vi "ADIS16448 Loop.vi"(8 "error in":errorcluster) -> ()   [LabVIEW 2019]
uses:
  Typedef/ADIS16448 Device Reference.ctl
  Typedef/ADIS16448 Hardware Configuration.ctl
  <vilib>/Rock Robotics/WPI/SPI/WPI_SPIMode.ctl
  <vilib>/Rock Robotics/SystemInterfaces/DIO/FPGA_DIOChannel.ctl
  <vilib>/Rock Robotics/SystemInterfaces/spilib/spi_bus.ctl
  Typedef/ADIS16448 Status.ctl
  Typedef/ADIS16448 Process.ctl
  Typedef/ADIS16448 Command Type.ctl
  <vilib>/Rock Robotics/SystemInterfaces/CounterEncoderSourceConvertion/FPGA_CounterEncoderSourceConvertionLVSourceType.ctl
  <vilib>/Rock Robotics/SystemInterfaces/DIO/FPGA_DIODigitalSourceChannel.ctl
  <vilib>/Rock Robotics/SystemInterfaces/AnalogTrigger/FPGA_AnalogTriggerIndex.ctl
  <vilib>/Rock Robotics/SystemInterfaces/AnalogTrigger/FPGA_AnalogTriggerOutType.ctl
  <vilib>/Rock Robotics/WPI/SPI/WPI_SPIDevRef.ctl
  Typedef/ADIS16448 Data.ctl
  Typedef/ADIS16448 Register.ctl
  <vilib>/Rock Robotics/WPI/Counter/WPI_CounterDigitalInputToDigitalSource.vi
panel:
  in  "Calibration Time":i32
  in  "ADIS16448DevRef":T1={"DevStatus"={"status"=FALSE, "code"=0, "source"=""}, "Hardware Config"={"SPI Clock Rate (Hz)"=1000000.0, "IMU SPI Mode (3)"=enum."Mode 3 (Clk Idle High,Sample on Trailing)", "IMU Reset Pin"=enum."SPI Port CS2", "IMU SPI Bus"=enum."SPI On-Board, CS0", "IMU Data Ready Pin"=enum."SPI Port CS1", "Stall Config"={"Pow2BytesPerRead"=255, "StallTicks"=640, "CsToSclkTicks"=5}, "IMU Status LED Pin"=enum."DIO MXP 9"}, "Calibration Complete"=refnum, "Last Value Reference"=refnum, "Sychronous Process VI"=refnum, "Cmd FIFO"=refnum, "Source"={"DevStatus"={"status"=FALSE, "code"=0, "source"=""}, "AnalogTriggerMode?"=FALSE, "DigitalMode"={"DIO Channel"=enum."Disabled"}, "AnalogTriggerMode"={"AnalogTriggerIndex"=enum."Trig 0", "OutputType"=enum."InWindow"}}, "IMU Status LED Pin"=enum."DIO MXP 9", "Calibration Time"=5}
  in  "Main Name":string
  # "I need to skip the first 6 points.\nDon't use pt-bt-pt to calc avg.\nPublish DC and RMS and CRC errors.\nAdd subVI to recalibrate.\nAdd back the Fuzing code"
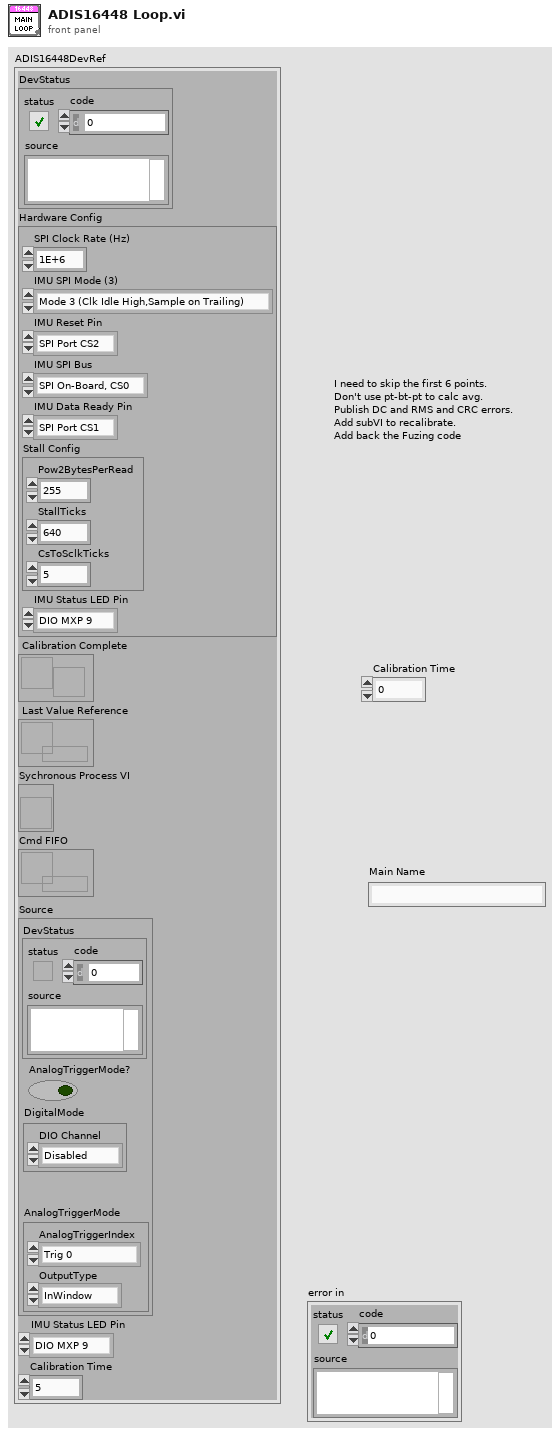
[diagram p1: front panel]
types:
  T1 = typedef "ADIS16448 Device Reference.ctl" = cluster{"DevStatus":errorcluster, "Hardware Config":T2, "Calibration Complete":refnum<notifier>, "Last Value Reference":refnum<data-value>, "Sychronous Process VI":T6, "Cmd FIFO":refnum<k33>, "Source":T7, "IMU Status LED Pin":T4, "Calibration Time":u32}
  T2 = typedef "ADIS16448 Hardware Configuration.ctl" = cluster{"SPI Clock Rate (Hz)":dbl, "IMU SPI Mode (3)":T3, "IMU Reset Pin":T4, "IMU SPI Bus":T5, "IMU Data Ready Pin":T4, "Stall Config":cluster{"Pow2BytesPerRead":u8, "StallTicks":u16, "CsToSclkTicks":u8}, "IMU Status LED Pin":T4}
  T3 = typedef "WPI_SPIMode.ctl" = enum16{"Mode 0 (Clk Idle Low,Sample on Leading)", "Mode 1 (Clk Idle Low,Sample on Trailing)", "Mode 2 (Clk Idle High,Sample on Leading)", "Mode 3 (Clk Idle High,Sample on Trailing)"}
  T4 = typedef "FPGA_DIOChannel.ctl" = enum8{"DIO 0", "DIO 1", "DIO 2", "DIO 3", "DIO 4", "DIO 5", "DIO 6", "DIO 7", "DIO 8", "DIO 9", "DIO MXP 0", "DIO MXP 1", "DIO MXP 2", "DIO MXP 3", "DIO MXP 4", "DIO MXP 5", "DIO MXP 6", "DIO MXP 7", "DIO MXP 8", "DIO MXP 9", "DIO MXP 10", "DIO MXP 11", "DIO MXP 12", "DIO MXP 13", "DIO MXP 14", "DIO MXP 15", "SPI Port CS1", "SPI Port CS2", "SPI Port CS3", "SPI Port MISO", "SPI Port MOSI", "Invalid"}
  T5 = typedef "spi_bus.ctl" = enum16{"SPI On-Board, CS0", "SPI On-Board, CS1", "SPI On-Board, CS2", "SPI On-Board, CS3", "SPI MXP", "Invalid"}
  T6 = typedef "ADIS16448 Process.ctl" = refnum<vi>
  T7 = typedef "FPGA_CounterEncoderSourceConvertionLVSourceType.ctl" = cluster{"DevStatus":errorcluster, "AnalogTriggerMode?":bool, "DigitalMode":cluster{"DIO Channel":T8}, "AnalogTriggerMode":cluster{"AnalogTriggerIndex":T9, "OutputType":T10}}
  T8 = typedef "FPGA_DIODigitalSourceChannel.ctl" = enum8{"DIO 0", "DIO 1", "DIO 2", "DIO 3", "DIO 4", "DIO 5", "DIO 6", "DIO 7", "DIO 8", "DIO 9", "DIO MXP 0", "DIO MXP 1", "DIO MXP 2", "DIO MXP 3", "DIO MXP 4", "DIO MXP 5", "DIO MXP 6", "DIO MXP 7", "DIO MXP 8", "DIO MXP 9", "DIO MXP 10", "DIO MXP 11", "DIO MXP 12", "DIO MXP 13", "DIO MXP 14", "DIO MXP 15", "SPI Port CS1", "SPI Port CS2", "SPI Port CS3", "SPI Port MISO", "SPI Port MOSI", "Disabled"}
  T9 = typedef "FPGA_AnalogTriggerIndex.ctl" = enum8{"Trig 0", "Trig 1", "Trig 2", "Trig 3", "Trig 4", "Trig 5", "Trig 6", "Trig 7", "Invalid"}
  T10 = typedef "FPGA_AnalogTriggerOutType.ctl" = enum16{"InWindow", "TriggerState", "Rising", "Falling"}
  T11 = cluster{"Gyro X":dbl, "Gyro Y":dbl, "Gyro Z":dbl}[]
  T12 = typedef "WPI_SPIDevRef.ctl" = cluster{"DevStatus":errorcluster, "Handle":i32, "SPI Bus":T5}
  T13 = cluster{"SPIDevRef":T12, "Data Counter":u16, "Digital Source":T7, "Bytes Per Sample":u32, "ADIS16448DevRef":T1, "TimeStampPrev":u32, "AutoSPI Active?":bool, "Offsets":cluster{"X":dbl, "Y":dbl, "Z":dbl}, "Offset Counter":i32, "Variance":cluster{"X":dbl, "Y":dbl, "Z":dbl}, "CRC Error Info":cluster{i32, i32}, "IMU Data":cluster{"Gyro Data":cluster{"X":dbl, "Y":dbl, "Z":dbl}, "Accel Data":cluster{"X":dbl, "Y":dbl, "Z":dbl}, "Mag Data":cluster{"X":dbl, "Y":dbl, "Z":dbl}, "Barometer":dbl, "Temperature":dbl}, "YPR Data Madgwick":cluster{"X":dbl, "Y":dbl, "Z":dbl}}
  T14 = cluster{"Gyro Data":cluster{"X":dbl, "Y":dbl, "Z":dbl}, "Accel Data":cluster{"X":dbl, "Y":dbl, "Z":dbl}, "Mag Data":cluster{"X":dbl, "Y":dbl, "Z":dbl}, "Barometer":dbl, "Temperature":dbl}
  T15 = typedef "ADIS16448 Status.ctl" = cluster{"Calibrated?":bool, "IMU Detected?":bool}
  T16 = typedef "ADIS16448 Register.ctl" = u8
  T17 = typedef "ADIS16448 Command Type.ctl" = cluster{"Command":enum16{"None", "Start Recal"}, "Data":u32}
  T18 = typedef "ADIS16448 Data.ctl" = cluster{"XAngle":dbl, "YAngle":dbl, "ZAngle":dbl}
  T19 = typedef "WPI_DigitalOutputDevRef.ctl" = cluster{"DIO Channel":T4, "DevStatus":errorcluster}
  T20 = typedef "WPI_DigitalInputDevRef.ctl" = cluster{"DevStatus":errorcluster, "DIO Channel":T4}
  T21 = cluster{T15, "Calibration Variance":cluster{"X Rotation":dbl, "Y Rotation":dbl, "Z Rotation":dbl}, "CRC Error Info":cluster{"Valid":i32, "Total":i32}, "IMU Data":cluster{"Gyro Data":cluster{"X":dbl, "Y":dbl, "Z":dbl}, "Accel Data":cluster{"X":dbl, "Y":dbl, "Z":dbl}, "Mag Data":cluster{"X":dbl, "Y":dbl, "Z":dbl}, "Barometer":dbl, "Temperature":dbl}, "Madgwick":cluster{"X":dbl, "Y":dbl, "Z":dbl}}
  T22 = cluster{"Pow2BytesPerRead":u8, "StallTicks":u16, "CsToSclkTicks":u8}
  T23 = cluster{cluster{"Gyro X":dbl, "Gyro Y":dbl, "Gyro Z":dbl}, cluster{"Accel X":dbl, "Accel Y":dbl, "Accel Z":dbl}, cluster{"Mag X":dbl, "Mag Y":dbl, "Mag Z":dbl}, "Baro":dbl, "Temp":dbl}
  T24 = cluster{"Gyro X":dbl, "Gyro Y":dbl, "Gyro Z":dbl}
  T25 = cluster{"variance":dbl, "variance":dbl, "variance":dbl}
  T26 = enum32{"Bad", "Idle", "Run top level", "Running"}
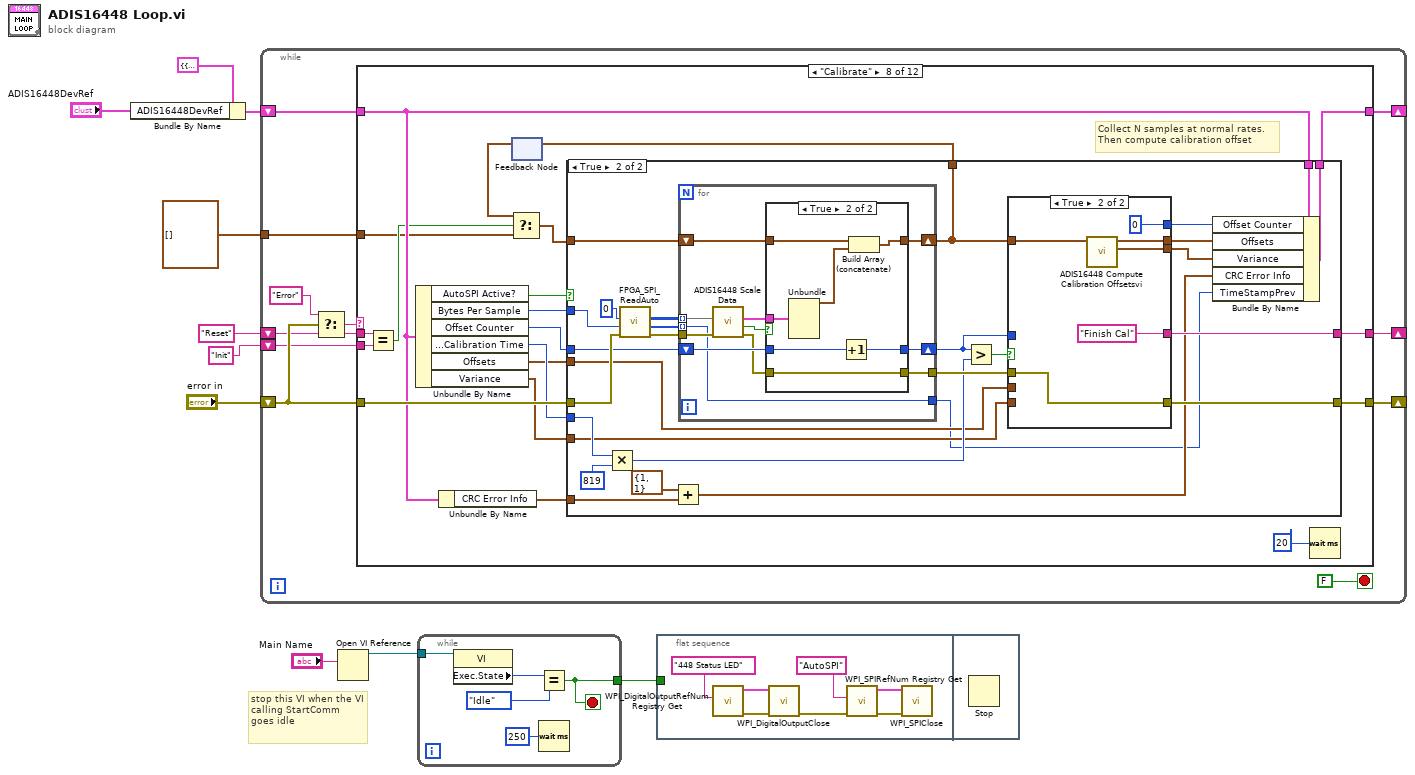
[diagram p0: block diagram]
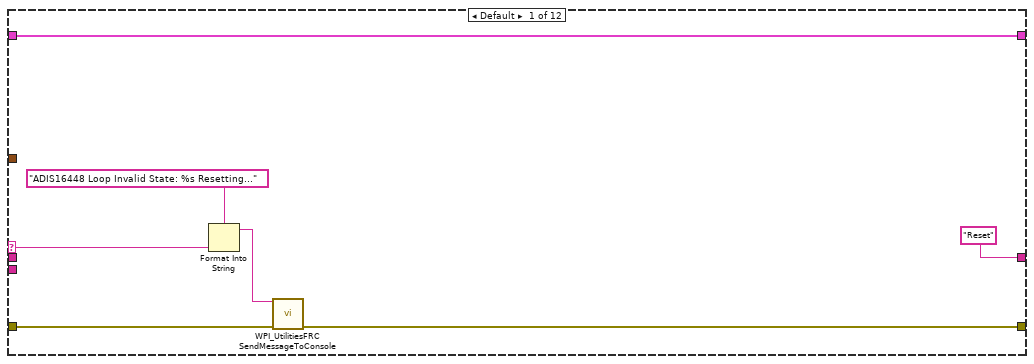
[diagram p2: hidden frame]
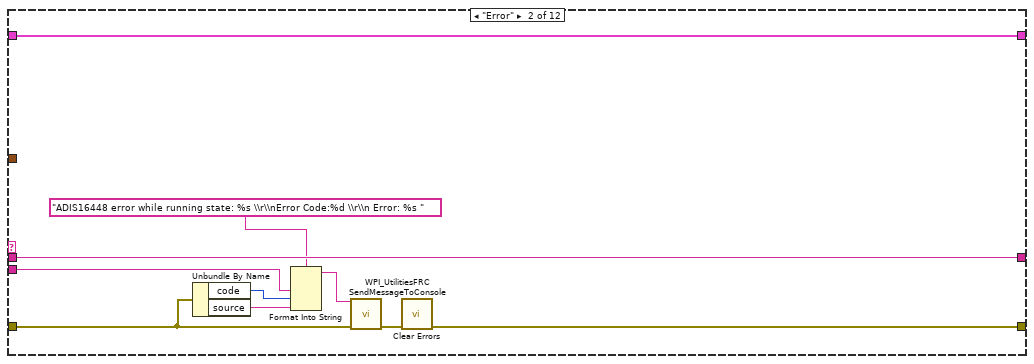
[diagram p3: hidden frame]
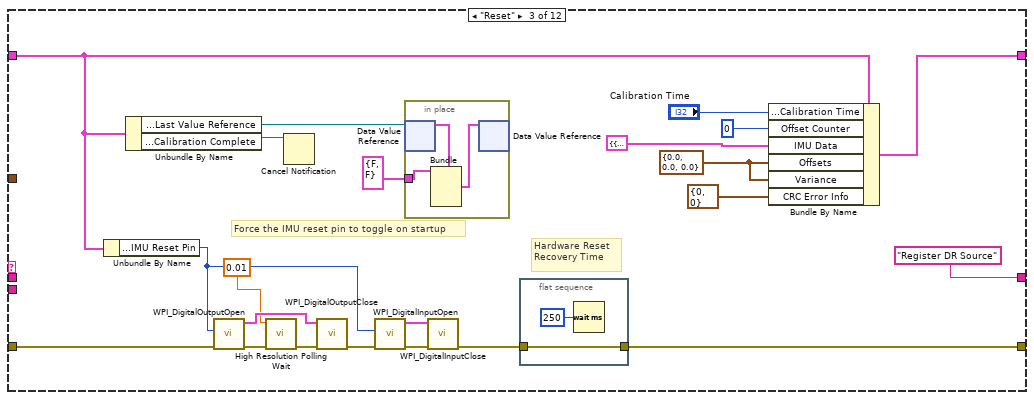
[diagram p4: hidden frame]
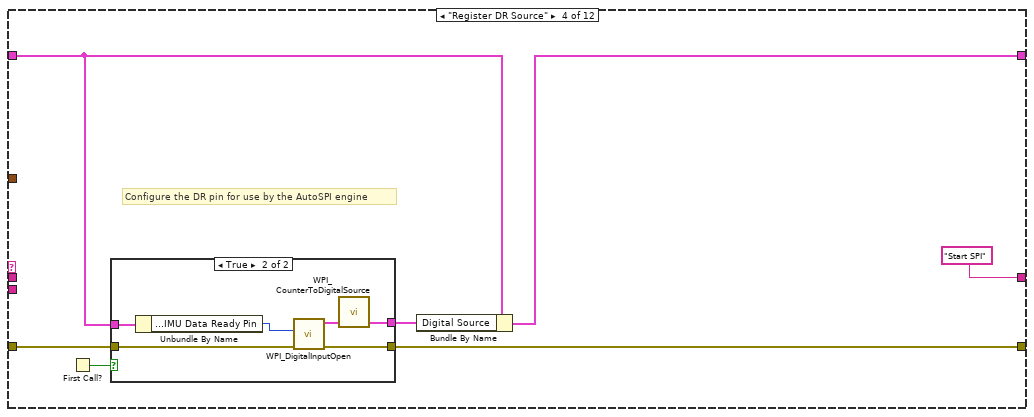
[diagram p5: hidden frame]
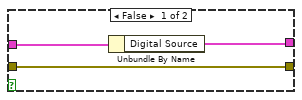
[diagram p6: hidden frame]
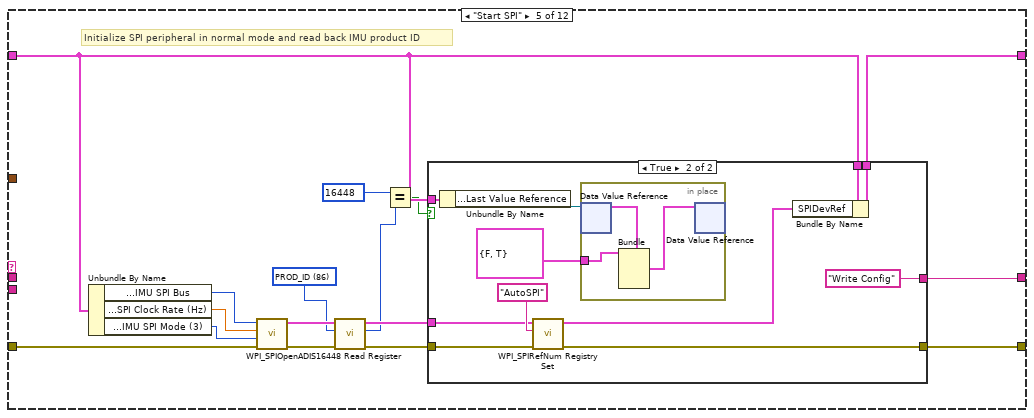
[diagram p7: hidden frame]
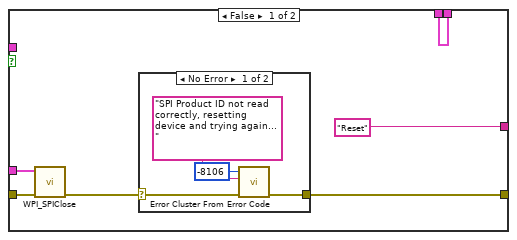
[diagram p8: hidden frame]
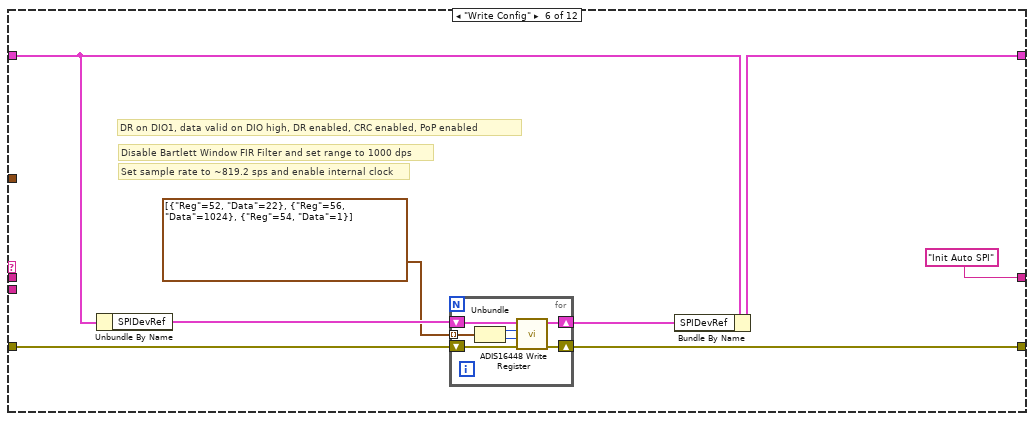
[diagram p10: hidden frame]
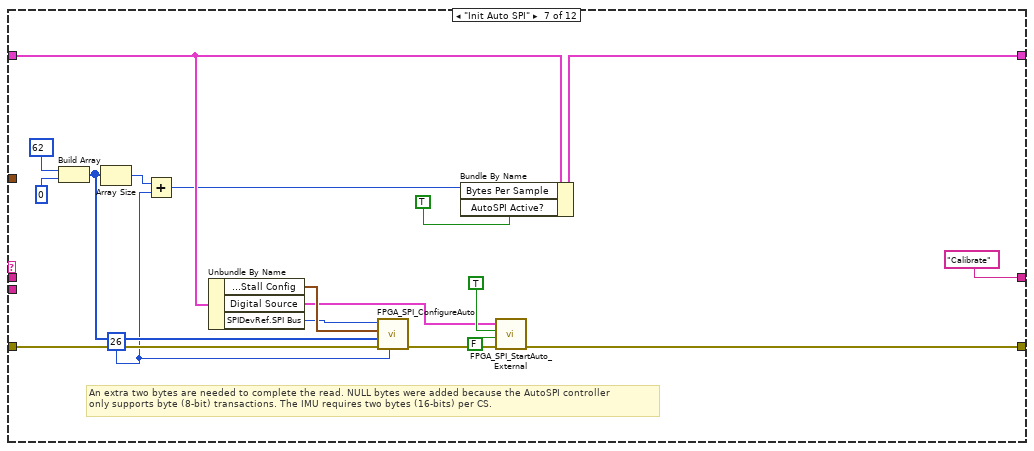
[diagram p11: hidden frame]
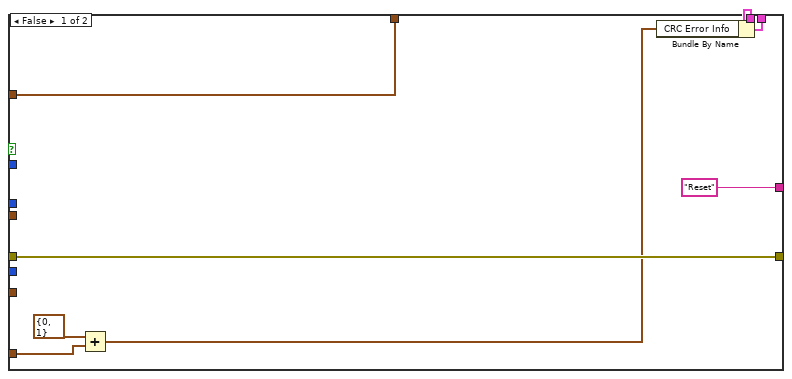
[diagram p12: hidden frame]
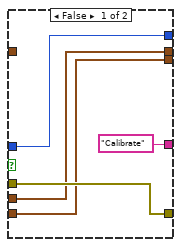
[diagram p13: hidden frame]
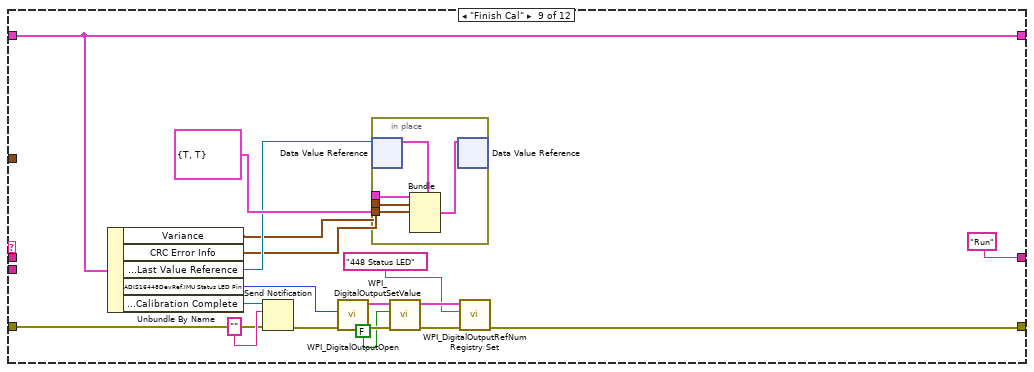
[diagram p15: hidden frame]
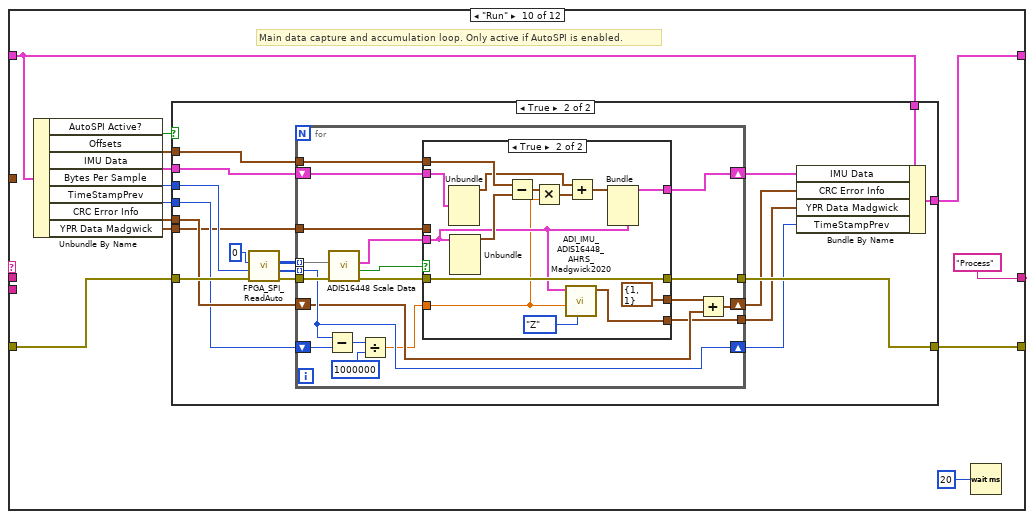
[diagram p16: hidden frame]
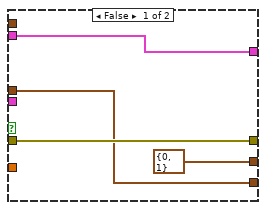
[diagram p18: hidden frame]
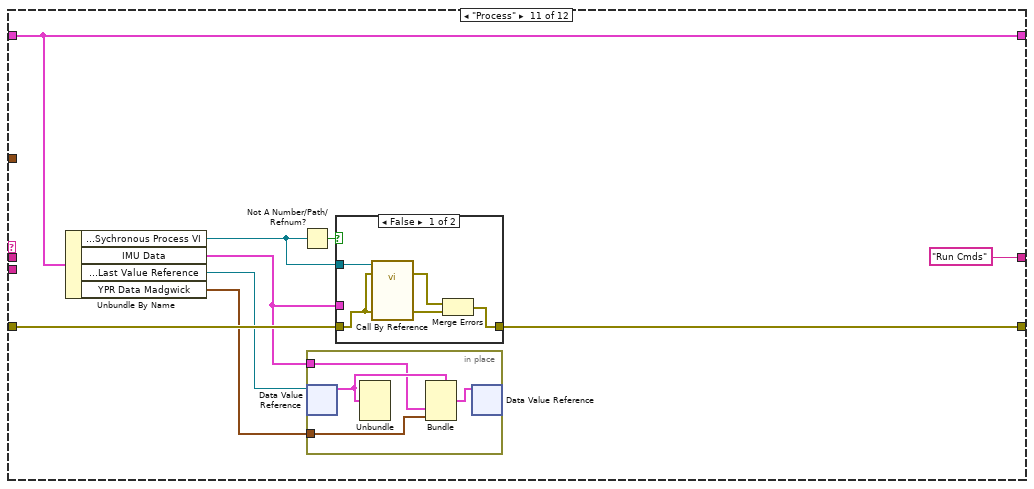
[diagram p19: hidden frame]
diagram:
  # "stop this VI when the VI calling StartComm goes idle"
  n1 = Bundle By Name(cluster=T13 {"SPIDevRef"={"DevStatus"={"status"=FALSE, "code"=0, "source"=""}, "Handle"=0, "SPI Bus"=enum."SPI On-Board, CS0"}, "Data Counter"=0, "Digital Source"={"DevStatus"={"status"=FALSE, "code"=0, "source"=""}, "AnalogTriggerMode?"=FALSE, "DigitalMode"={"DIO Channel"=enum."DIO 1"}, "AnalogTriggerMode"={"AnalogTriggerIndex"=enum."Trig 0", "OutputType"=enum."InWindow"}}, "Bytes Per Sample"=0, "ADIS16448DevRef"={"DevStatus"={"status"=FALSE, "code"=0, "source"=""}, "Hardware Config"={"SPI Clock Rate (Hz)"=1000000.0, "IMU SPI Mode (3)"=enum."Mode 3 (Clk Idle High,Sample on Trailing)", "IMU Reset Pin"=enum."SPI Port CS2", "IMU SPI Bus"=enum."SPI On-Board, CS0", "IMU Data Ready Pin"=enum."SPI Port CS1", "Stall Config"={"Pow2BytesPerRead"=255, "StallTicks"=640, "CsToSclkTicks"=5}, "IMU Status LED Pin"=enum."DIO MXP 9"}, "Calibration Complete"=refnum, "Last Value Reference"=refnum, "Sychronous Process VI"=refnum, "Cmd FIFO"=refnum, "Source"={"DevStatus"={"status"=FALSE, "code"=0, "source"=""}, "AnalogTriggerMode?"=FALSE, "DigitalMode"={"DIO Channel"=enum."Disabled"}, "AnalogTriggerMode"={"AnalogTriggerIndex"=enum."Trig 0", "OutputType"=enum."InWindow"}}, "IMU Status LED Pin"=enum."DIO MXP 9", "Calibration Time"=5}, "TimeStampPrev"=0, "AutoSPI Active?"=TRUE, "Offsets"={"X"=0.0, "Y"=0.0, "Z"=0.0}, "Offset Counter"=0, "Variance"={"X"=0.0, "Y"=0.0, "Z"=0.0}, "CRC Error Info"={0, 0}, "IMU Data"={"Gyro Data"={"X"=0.0, "Y"=0.0, "Z"=0.0}, "Accel Data"={"X"=0.0, "Y"=0.0, "Z"=0.0}, "Mag Data"={"X"=0.0, "Y"=0.0, "Z"=0.0}, "Barometer"=0.0, "Temperature"=0.0}, "YPR Data Madgwick"={"X"=0.0, "Y"=0.0, "Z"=0.0}}, "ADIS16448DevRef"="ADIS16448DevRef") -> (w6:T13)
  n2 = while {
    shift-right: [w17] -> _
    shift-left: "Reset" -> [w14]
    shift-right: [w19] -> _
    shift-left: w6 -> [w20]
    shift-right: [w18] -> _
    shift-left: "error in" -> [w16]
    shift-left: "Init" -> [w12]
    tunnel: T11 [] ("f") -> [w11]
    stop <- FALSE stop-if-true
    n3 = Select(t="Error", s=w16, f=w14) -> (s? t:f=w15:string)
    n4 = case shown="\"Calibrate\"" w15 {
      selector: w15 -> [w27 _ _ _ _ _ _ _ _ _ _ _]
      tunnel: w20 -> [w28 w38 w57 w67 w84 w125 w150 w161 w244 w274 w344 w358]
      tunnel: [w28 w38 w56 w71 w83 w124 w149 w172 w244 w278 w344 w363] -> w19
      tunnel: w16 -> [w26 w34 w50 w70 w97 w128 w154 w174 w258 w277 w343 w365]
      tunnel: [w25 w35 w59 w68 w92 w127 w138 w173 w251 w276 w342 w364] -> w18
      tunnel: ["Reset" w37 "Register DR Source" "Start SPI" w93 "Init Auto SPI" "Calibrate" w168 "Run" "Process" "Run Cmds" w356] -> w17
      tunnel: w14 -> [_ w37 _ _ _ _ _ w166 _ _ _ _]
      tunnel: w12 -> [_ w30 _ _ _ _ _ w165 _ _ _ _]
      tunnel: w11 -> [_ _ _ _ _ _ _ w156 _ _ _ _]
      frame Default {
        n5 = Format Into String(format string="ADIS16448 Loop Invalid State: %s Resetting...", w27) -> (resulting string=w24:string)  [unwired: 2 in, 1 out]
        n6 = call <vilib>:"WPI_UtilitiesFRC SendMessageToConsole.vi"("Message"=w24, "error in (no error)"=w26) -> ("error out"=w25:errorcluster)  [unwired: 13 in]
      }
      frame "Error" {
        n7 = Unbundle By Name(w34) -> ("code"=w32:i32, "source"=w31:string)
        n8 = Format Into String(format string="ADIS16448 error while running state: %s \\r\\nError Code:%d \\r\\n Error: %s ", w30, w32, w31) -> (resulting string=w33:string)  [unwired: 2 in, 1 out]
        n9 = call <vilib>:"WPI_UtilitiesFRC SendMessageToConsole.vi"("Message"=w33, "error in (no error)"=w34) -> ("error out"=w36:errorcluster)  [unwired: 13 in]
        n10 = call <vilib>:"Clear Errors.vi"("error in (no error)"=w36) -> ("error out"=w35:errorcluster)  [unwired: 5 in, 1 out]
      }
      frame "Reset" {
        w41 = T18 {"XAngle"=0.0, "YAngle"=0.0, "ZAngle"=0.0} ("element")
        # "Hardware Reset Recovery Time"
        # "Force the IMU reset pin to toggle on startup"
        n11 = Unbundle By Name(w57) -> ("ADIS16448DevRef.Hardware Config.IMU Reset Pin"=w46:T4)
        n12 = Unbundle By Name(w57) -> ("ADIS16448DevRef.Last Value Reference"=w43:refnum<data-value>, "ADIS16448DevRef.Calibration Complete"=w58:refnum<notifier>)
        n13 = call <vilib>:"WPI_DigitalOutputOpen.vi"("error in (no error)"=w50, "DIO Channel"=w46) -> ("error out"=w48:errorcluster, "DigitalOutputDevRef"=w55:T19)  [unwired: 8 in]
        n14 = call <vilib>:"High Resolution Polling Wait.vi"("error in (no error)"=w48, "seconds to wait"=0.01) -> ("error out"=w49:errorcluster)  [unwired: 9 in]
        n15 = Cancel Notification(0:w58) -> ()  [unwired: 1 in, 3 out]
        n16 = call <vilib>:"WPI_DigitalOutputClose.vi"("error in (no error)"=w49, "DigitalOutputDevRef"=w55) -> ("error out"=w52:errorcluster)  [unwired: 9 in]
        n17 = call <vilib>:"WPI_DigitalInputOpen.vi"("error in (no error)"=w52, "DIO Channel"=w46) -> ("error out"=w53:errorcluster, "DigitalInputDevRef"=w54:T20)  [unwired: 8 in]
        n18 = in-place {
          in-place-border: T15 {"Calibrated?"=FALSE, "IMU Detected?"=FALSE} ("element") -> [w61]
          n19 = in-place-dvr #1(w43) -> (w62:T21)  [unwired: 1 out]
          n20 = Bundle(cluster=w62, w61) -> (w63:T21)  [unwired: 4 in]
          n21 = in-place-dvr #1(w63) -> ()  [unwired: 2 out]
        }
        n22 = call <vilib>:"WPI_DigitalInputClose.vi"("error in (no error)"=w53, "DigitalInputDevRef"=w54) -> ("error out"=w51:errorcluster)  [unwired: 9 in]
        n23 = flat-sequence {
          tunnel: [w65] -> w59
          tunnel: w51 -> [w65]
          frame #0 {
            n24 = Wait (ms)(milliseconds to wait=u32 250) -> ()  [unwired: 1 out]
          }
        }
        n25 = Bundle By Name(cluster=w57, "ADIS16448DevRef.Calibration Time"="Calibration Time", "Offset Counter"=0, "IMU Data"=T14 {"Gyro Data"={"X"=0.0, "Y"=0.0, "Z"=0.0}, "Accel Data"={"X"=0.0, "Y"=0.0, "Z"=0.0}, "Mag Data"={"X"=0.0, "Y"=0.0, "Z"=0.0}, "Barometer"=0.0, "Temperature"=0.0}, "Offsets"=w41, "Variance"=w41, "CRC Error Info"=cluster{i32, i32} {0, 0}) -> (w56:T13)
      }
      frame "Register DR Source" {
        # "Configure the DR pin for use by the AutoSPI engine"
        n26 = First Call?() -> (First Call?: T/F=w66:bool)
        n27 = case shown="True" w66 {
          tunnel: w70 -> [w73 w81]
          tunnel: w67 -> [w75 w79]
          tunnel: [w74 w77] -> w69
          tunnel: [w73 w76] -> w68
          frame False {
            n28 = Unbundle By Name(w75) -> ("Digital Source"=w74:T7)
          }
          frame True {
            n29 = Unbundle By Name(w79) -> ("ADIS16448DevRef.Hardware Config.IMU Data Ready Pin"=w78:T4)
            n30 = call <vilib>:"WPI_DigitalInputOpen.vi"("error in (no error)"=w81, "DIO Channel"=w78) -> ("error out"=w76:errorcluster, "DigitalInputDevRef"=w80:T20)  [unwired: 8 in]
            n31 = call-poly <vilib>:"WPI_CounterToDigitalSource.vi"("DigitalInputDevRef"=w80) -> ("Digital Source"=w77:T7)  [unwired: 6 in]
          }
        }
        n32 = Bundle By Name(cluster=w67, "Digital Source"=w69) -> (w71:T13)
      }
      frame "Start SPI" {
        w88 = T16 86 items=["FLASH_CNT"=0, "Reserved 1"=2, "XGYRO_OUT"=4, "YGYRO_OUT"=6, "ZGYRO_OUT"=8, "XACCL_OUT"=10, "YACCL_OUT"=12, "ZACCL_OUT"=14, "XMAGN_OUT"=16, "YMAGN_OUT"=18, "ZMAGN_OUT"=20, "BARO_OUT"=22, "TEMP_OUT"=24, "XGYRO_OFF"=26, "YGYRO_OFF"=28, "ZGYRO_OFF"=30, "XACCL_OFF"=32, "YACCL_OFF"=34, "ZACCL_OFF"=36, "XMAGN_HIC"=38, "YMAGN_HIC"=40, "ZMAGN_HIC"=42, "XMAGN_SIC"=44, "YMAGN_SIC"=46, "ZMAGN_SIC"=48, "GPIO_CTRL"=50, "MSC_CTRL"=52, "SMPL_PRD"=54, "SENS_AVG"=56, "SEQ_CNT"=58, "DIAG_STAT"=60, "GLOB_CMD"=62, "ALM_MAG1"=64, "ALM_MAG2"=66, "ALM_SMPL1"=68, "ALM_SMPL2"=70, "ALM_CTRL"=72, "Reserved 2"=74, "Reserved 3"=76, "Reserved 4"=78, "Reserved 5"=80, "LOT_ID1"=82, "LOT_ID2"=84, "PROD_ID"=86, "SERIAL_NUM"=88] ("ADIS16448 Register")
        # "Initialize SPI peripheral in normal mode and read back IMU product ID"
        n33 = Unbundle By Name(w84) -> ("ADIS16448DevRef.Hardware Config.IMU SPI Bus"=w94:T5, "ADIS16448DevRef.Hardware Config.SPI Clock Rate (Hz)"=w95:dbl, "ADIS16448DevRef.Hardware Config.IMU SPI Mode (3)"=w96:T3)
        n34 = call <vilib>:"WPI_SPIOpen.vi"("error in"=w97, "Mode (3)"=w96, "Clock Rate (Hz)"=w95, "SPI Bus"=w94) -> ("error out"=w91:errorcluster, "SPIDevRef"=w90:T12)  [unwired: 6 in]
        n35 = call "ADIS16448 Read Register.vi"("error in (no error)"=w91, "ADIS16448 Register"=w88, "SPIDevRef in"=w90) -> ("error out"=w86:errorcluster, "Register Value"=w85:u16, "SPIDevRef out"=w87:T12)  [unwired: 6 in]
        n36 = Equal?(x=u16 16448 ("y"), y=w85) -> (x = y?=w82:bool)
        n37 = case shown="True" w82 {
          tunnel: ["Reset" "Write Config"] -> w93
          tunnel: w84 -> [w102 w118]
          tunnel: [w102 w117] -> w83
          tunnel: [w101 w112] -> w92
          tunnel: w86 -> [w100 w113]
          tunnel: w87 -> [w99 w114]
          tunnel: w84 -> [_ w111]
          frame False {
            n38 = call <vilib>:"WPI_SPIClose.vi"("error in (no error)"=w100, "SPIDevRef"=w99) -> ("error out"=w98:errorcluster)  [unwired: 9 in]
            n39 = case shown="No Error" w98 {
              selector: w98 -> [w106 w108]
              tunnel: [w107 w108] -> w101
              frame No Error {
                n40 = call <vilib>:"Error Cluster From Error Code.vi"("error in (no error)"=w106, "error message (\"\")"="SPI Product ID not read correctly, resetting device and trying again..." ("error message (\"\")"), "error code (0)"=-8106) -> ("error out"=w107:errorcluster)  [unwired: 6 in]
              }
              frame Error {
              }
            }
          }
          frame True {
            n41 = Unbundle By Name(w111) -> ("ADIS16448DevRef.Last Value Reference"=w109:refnum<data-value>)
            n42 = call <vilib>:"WPI_SPIRefNum Registry Set.vi"("error in (no error)"=w113, "refnum name"="AutoSPI", "SPIDevRef"=w114) -> ("error out"=w112:errorcluster, "SPIDevRef"=w116:T12)  [unwired: 7 in]
            n43 = in-place {
              in-place-border: T15 {"Calibrated?"=FALSE, "IMU Detected?"=TRUE} ("element") -> [w120]
              n44 = in-place-dvr #2(w109) -> (w121:T21)  [unwired: 1 out]
              n45 = Bundle(cluster=w121, w120) -> (w122:T21)  [unwired: 4 in]
              n46 = in-place-dvr #2(w122) -> ()  [unwired: 2 out]
            }
            n47 = Bundle By Name(cluster=w118, "SPIDevRef"=w116) -> (w117:T13)
          }
        }
      }
      frame "Write Config" {
        # "DR on DIO1, data valid on DIO high, DR enabled, CRC enabled, PoP enabled"
        # "Set sample rate to ~819.2 sps and enable internal clock"
        # "Disable Bartlett Window FIR Filter and set range to 1000 dps"
        n48 = Unbundle By Name(w125) -> ("SPIDevRef"=w129:T12)
        n49 = for {
          tunnel: cluster{"Reg":T16, "Data":u16}[] [{"Reg"=52, "Data"=22}, {"Reg"=56, "Data"=1024}, {"Reg"=54, "Data"=1}] -> [w137] mode=indexing
          shift-right: [w133] -> w127
          shift-left: w128 -> [w132]
          shift-right: [w131] -> w123
          shift-left: w129 -> [w134]
          n50 = Unbundle(w137) -> ("Reg"=w136:T16, "Data"=w135:u16)
          n51 = call "ADIS16448 Write Register.vi"("error in (no error)"=w132, "Data"=w135, "Register"=w136, "SPIDevRef in"=w134) -> ("error out"=w133:errorcluster, "SPIDevRef out"=w131:T12)  [unwired: 6 in]
        }
        n52 = Bundle By Name(cluster=w125, "SPIDevRef"=w123) -> (w124:T13)
      }
      frame "Init Auto SPI" {
        w139 = u8 26 ("dimension size")
        # "An extra two bytes are needed to complete the read. NULL bytes were added because the AutoSPI controller \nonly supports byte (8-bit) transactions. The IMU requires two bytes (16-bits) per CS."
        n53 = Build Array(u8 62 ("hi"), u8 0 ("element")) -> (w140:u8[])
        n54 = Array Size(array=w140) -> (size(s)=w144:i32)
        n55 = Add(x=w144, y=w139) -> (x+y=w141:i32)
        n56 = Unbundle By Name(w150) -> ("ADIS16448DevRef.Hardware Config.Stall Config"=w148:T22, "Digital Source"=w146:T7, "SPIDevRef.SPI Bus"=w145:T5)
        n57 = call <vilib>:"FPGA_SPI_ConfigureAuto.vi"("SPI Auto Zero Byte Count"=w139, "error in"=w154, "SPI Auto TX Byte Array"=w140, "Stall Config"=w148, "SPI Bus"=w145) -> ("error out"=w153:errorcluster)  [unwired: 6 in]
        n58 = Bundle By Name(cluster=w150, "Bytes Per Sample"=w141, "AutoSPI Active?"=TRUE) -> (w149:T13)
        n59 = call <vilib>:"FPGA_SPI_StartAuto_External.vi"("error in (no error)"=w153, "Falling Edge"=FALSE, "Rising Edge"=TRUE, "Source"=w146) -> ("error out"=w138:errorcluster)  [unwired: 7 in]
      }
      frame "Calibrate" {
        # "Collect N samples at normal rates.\nThen compute calibration offset"
        n60 = Equal?(x=w166, y=w165) -> (x = y?=w159:bool)
        n61 = Unbundle By Name(w161) -> ("AutoSPI Active?"=w175:bool, "Bytes Per Sample"=w171:u32, "Offset Counter"=w170:i32, "ADIS16448DevRef.Calibration Time"=w169:u32, "Offsets"=w164:cluster{"X":dbl, "Y":dbl, "Z":dbl}, "Variance"=w162:cluster{"X":dbl, "Y":dbl, "Z":dbl})
        n62 = Unbundle By Name(w161) -> ("CRC Error Info"=w160:cluster{i32, i32})
        n63 = feedback #3() -> (w158:T11)  [unwired: 1 in]
        n64 = Select(t=w158, s=w159, f=w156) -> (s? t:f=w157:T11)
        n65 = case shown="True" w175 {
          tunnel: [w178 w211] -> w172
          tunnel: w174 -> [w183 w206]
          tunnel: [w183 w197] -> w173
          tunnel: w161 -> [w177 w207]
          tunnel: w171 -> [_ w204]
          tunnel: w170 -> [_ w201]
          tunnel: w169 -> [_ w202]
          tunnel: ["Reset" w198] -> w168
          tunnel: w164 -> [_ w194]
          tunnel: [w181 w188] -> w163
          tunnel: w157 -> [w181 w187]
          tunnel: w162 -> [_ w193]
          tunnel: w160 -> [w180 w192]
          frame False {
            n66 = Add(x=cluster{i32, i32} {0, 1}, y=w180) -> (x+y=w176:cluster{i32, i32})
            n67 = Bundle By Name(cluster=w177, "CRC Error Info"=w176) -> (w178:T13)
          }
          frame True {
            n68 = Multiply(x=w202, y=819) -> (x*y=w195:u32)
            n69 = call <vilib>:"FPGA_SPI_ReadAuto.vi"("error in (no error)"=w206, "Bytes per Sample"=w204, "Samples to Read"=u32 0) -> ("error out"=w205:errorcluster, "Timestamps"=w208:u32[], "Data"=w209:u8[][])  [unwired: 6 in]
            n70 = Add(x=cluster{i32, i32} {1, 1}, y=w192) -> (x+y=w190:cluster{i32, i32})
            n71 = for {
              tunnel: w209 -> [w233] mode=indexing
              tunnel: w208 -> [w223] mode=indexing
              tunnel: w205 -> [w232]
              tunnel: [w227] -> w196
              shift-right: [w228] -> w199
              shift-left: w201 -> [w229]
              shift-right: [w224] -> w188
              shift-left: w187 -> [w225]
              tunnel: [w223] -> w189
              n72 = call "ADIS16448 Scale Data.vi"("error in (no error)"=w232, "New Data In"=w233) -> ("error out"=w226:errorcluster, "Data Good?"=w231:bool, "Data"=w230:T23)  [unwired: 7 in]
              n73 = case shown="True" w231 {
                tunnel: w230 -> [_ w240]
                tunnel: w229 -> [w236 w242]
                tunnel: [w236 w241] -> w228
                tunnel: [w235 w243] -> w227
                tunnel: w226 -> [w235 w243]
                tunnel: w225 -> [w234 w239]
                tunnel: [w234 w238] -> w224
                frame False {
                }
                frame True {
                  n74 = Unbundle(w240) -> (w237:T24)  [unwired: 4 out]
                  n75 = Increment(x=w242) -> (x+1=w241:i32)
                  n76 = Build Array (concatenate)(w239, w237) -> (w238:T11)
                }
              }
            }
            n77 = Greater?(x=w199, y=w195) -> (0:w200:bool)
            n78 = case shown="True" w200 {
              tunnel: w199 -> [w214 _]
              tunnel: ["Calibrate" "Finish Cal"] -> w198
              tunnel: [w215 w221] -> w197
              tunnel: w196 -> [w215 w221]
              tunnel: w188 -> [_ w220]
              tunnel: w194 -> [w213 _]
              tunnel: w193 -> [w212 _]
              tunnel: [w212 w219] -> w186
              tunnel: [w213 w218] -> w185
              tunnel: [w214 0 ("Offset Counter")] -> w184
              frame False {
              }
              frame True {
                n79 = call "ADIS16448 Compute Calibration Offsetsvi.vi"("Array"=w220) -> ("Variance"=w219:T25, "DC value"=w218:cluster{"mean":dbl, "mean":dbl, "mean":dbl})  [unwired: 9 in]
              }
            }
            n80 = Bundle By Name(cluster=w207, "Offset Counter"=w184, "Offsets"=w185, "Variance"=w186, "CRC Error Info"=w190, "TimeStampPrev"=w189) -> (w211:T13)
          }
        }
        n81 = feedback-in #3(w163) -> ()
        n82 = Wait (ms)(milliseconds to wait=u32 20) -> ()  [unwired: 1 out]
      }
      frame "Finish Cal" {
        n83 = Unbundle By Name(w244) -> ("Variance"=w245:cluster{"X":dbl, "Y":dbl, "Z":dbl}, "CRC Error Info"=w246:cluster{i32, i32}, "ADIS16448DevRef.Last Value Reference"=w247:refnum<data-value>, "ADIS16448DevRef.IMU Status LED Pin"=w248:T4, "ADIS16448DevRef.Calibration Complete"=w260:refnum<notifier>)
        n84 = Send Notification(notification="", notifier=w260, error in (no error)=w258) -> (error out=w252:errorcluster)  [unwired: 1 out]
        n85 = call <vilib>:"WPI_DigitalOutputOpen.vi"("error in (no error)"=w252, "DIO Channel"=w248) -> ("error out"=w257:errorcluster, "DigitalOutputDevRef"=w256:T19)  [unwired: 8 in]
        n86 = in-place {
          in-place-border: T15 {"Calibrated?"=TRUE, "IMU Detected?"=TRUE} ("element") -> [w264]
          in-place-border: w246 -> [w262]
          in-place-border: w245 -> [w263]
          n87 = in-place-dvr #4(w247) -> (w265:T21)  [unwired: 1 out]
          n88 = Bundle(cluster=w265, w264, "Calibration Variance"=w263, "CRC Error Info"=w262) -> (w266:T21)  [unwired: 2 in]
          n89 = in-place-dvr #4(w266) -> ()  [unwired: 2 out]
        }
        n90 = call <vilib>:"WPI_DigitalOutputSetValue.vi"("error in (no error)"=w257, "Value"=FALSE, "DigitalOutputDevRef"=w256) -> ("error out"=w255:errorcluster, "DigitalOutputDevRef"=w254:T19)  [unwired: 7 in]
        n91 = call <vilib>:"WPI_DigitalOutputRefNum Registry Set.vi"("error in (no error)"=w255, "refnum name"="448 Status LED", "DigitalOutputDevRef"=w254) -> ("error out"=w251:errorcluster)  [unwired: 7 in, 1 out]
      }
      frame "Run" {
        # "Main data capture and accumulation loop. Only active if AutoSPI is enabled."
        n92 = Unbundle By Name(w274) -> ("AutoSPI Active?"=w273:bool, "Offsets"=w272:cluster{"X":dbl, "Y":dbl, "Z":dbl}, "IMU Data"=w271:T14, "Bytes Per Sample"=w270:u32, "TimeStampPrev"=w268:u32, "CRC Error Info"=w269:cluster{i32, i32}, "YPR Data Madgwick"=w267:cluster{"X":dbl, "Y":dbl, "Z":dbl})
        n93 = case shown="True" w273 {
          tunnel: [w280 w299] -> w278
          tunnel: w277 -> [w281 w294]
          tunnel: [w281 w292] -> w276
          tunnel: w274 -> [w280 w295]
          tunnel: w272 -> [_ w289]
          tunnel: w271 -> [_ w288]
          tunnel: w270 -> [_ w287]
          tunnel: w269 -> [_ w286]
          tunnel: w268 -> [_ w285]
          tunnel: w267 -> [_ w283]
          frame False {
          }
          frame True {
            n94 = call <vilib>:"FPGA_SPI_ReadAuto.vi"("error in (no error)"=w294, "Bytes per Sample"=w287, "Samples to Read"=u32 0) -> ("error out"=w293:errorcluster, "Timestamps"=w296:u32[], "Data"=w297:u8[][])  [unwired: 6 in]
            n95 = for {
              tunnel: w297 -> [w317] mode=indexing
              tunnel: w296 -> [w308] mode=indexing
              shift-right: [w312] -> w290
              shift-left: w288 -> [w311]
              shift-right: [w308] -> w282
              shift-left: w285 -> [w318]
              tunnel: w293 -> [w316]
              tunnel: w289 -> [w315]
              tunnel: [w309] -> w292
              shift-right: [w305] -> w291
              shift-left: w286 -> [w306]
              tunnel: [w302] -> w284
              tunnel: w283 -> [w300]
              n96 = Subtract(x=w308, y=w318) -> (x-y=w314:u32)
              n97 = call "ADIS16448 Scale Data.vi"("error in (no error)"=w316, "New Data In"=w317) -> ("error out"=w310:errorcluster, "Data Good?"=w301:bool, "Data"=w303:T23)  [unwired: 7 in]
              n98 = Divide(x=w314, y=u32 1000000) -> (x/y=w304:dbl)
              n99 = case shown="True" w301 {
                tunnel: w303 -> [_ w324]
                tunnel: w315 -> [_ w332]
                tunnel: w304 -> [_ w323]
                tunnel: [w322 w327] -> w312
                tunnel: w311 -> [w322 w328]
                tunnel: w310 -> [w321 w334]
                tunnel: [w321 w334] -> w309
                tunnel: [cluster{i32, i32} {0, 1} cluster{i32, i32} {1, 1}] -> w307
                tunnel: [w319 w325] -> w302
                tunnel: w300 -> [w319 _]
                frame False {
                }
                frame True {
                  n100 = Unbundle(w328) -> ("Gyro Data"=w330:cluster{"X":dbl, "Y":dbl, "Z":dbl})  [unwired: 4 out]
                  n101 = Unbundle(w324) -> (w333:T24)  [unwired: 4 out]
                  n102 = Subtract(x=w332, y=w333) -> (x-y=w336:cluster{dbl, dbl, dbl})
                  n103 = Multiply(x=w336, y=w323) -> (x*y=w335:cluster{dbl, dbl, dbl})
                  n104 = call "ADI_IMU_ADIS16448_AHRS_Madgwick2020.vi"("Yaw Axis"=enum16{"X", "Y", "Z"}."Z", "delta t"=w323, "Data 2"=w324) -> ("Output"=w325:cluster{"Pitch":dbl, "Roll":dbl, "Yaw":dbl})  [unwired: 8 in]
                  n105 = Add(x=w330, y=w335) -> (x+y=w329:cluster{dbl, dbl, dbl})
                  n106 = Bundle(cluster=w324, w329) -> (w327:T23)  [unwired: 4 in]
                }
              }
              n107 = Add(x=w307, y=w306) -> (x+y=w305:cluster{i32, i32})
            }
            n108 = Bundle By Name(cluster=w295, "IMU Data"=w290, "CRC Error Info"=w291, "YPR Data Madgwick"=w284, "TimeStampPrev"=w282) -> (w299:T13)
          }
        }
        n109 = Wait (ms)(milliseconds to wait=u32 20) -> ()  [unwired: 1 out]
      }
      frame "Process" {
        n110 = Unbundle By Name(w344) -> ("ADIS16448DevRef.Sychronous Process VI"=w340:T6, "IMU Data"=w339:T14, "ADIS16448DevRef.Last Value Reference"=w338:refnum<data-value>, "YPR Data Madgwick"=w337:cluster{"X":dbl, "Y":dbl, "Z":dbl})
        n111 = Not A Number/Path/Refnum?(number/path/refnum=w340) -> (NaN/Path/Refnum?=w341:bool)
        n112 = in-place {
          in-place-border: w339 -> [w347]
          in-place-border: w337 -> [w346]
          n113 = in-place-dvr #5(w338) -> (w348:T21)  [unwired: 1 out]
          n114 = Unbundle(w348) -> ()  [unwired: 5 out]
          n115 = Bundle(cluster=w348, "IMU Data"=w347, "Madgwick"=w346) -> (w349:T21)  [unwired: 3 in]
          n116 = in-place-dvr #5(w349) -> ()  [unwired: 2 out]
        }
        n117 = case shown="False" w341 {
          tunnel: w343 -> [w351 w355]
          tunnel: w339 -> [_ _]
          tunnel: [w354 w355] -> w342
          tunnel: w340 -> [w350 _]
          frame False {
            n118 = call-by-ref "?"(reference=w350, error in=w351, 8:"error in (no error)"=w351) -> (error out=w352:errorcluster, 0:"error out"=w353:errorcluster)  [unwired: 10 in, 1 out]
            n119 = Merge Errors(w352, w353) -> (w354:errorcluster)
          }
          frame True {
          }
        }
      }
      frame "Run Cmds" {
        n120 = Unbundle By Name(w358) -> ("ADIS16448DevRef.Cmd FIFO"=w366:refnum<k33>)
        n121 = Unbundle By Name(w358) -> ("ADIS16448DevRef.Last Value Reference"=w361:refnum<data-value>, "ADIS16448DevRef.Calibration Complete"=w362:refnum<notifier>)
        n122 = RT FIFO Read(0:w366, 1:T17 {"Command"=enum."None", "Data"=0} ("element")) -> (9:w360:T17)  [unwired: 2 in, 4 out]
        n123 = Unbundle(w360) -> ("Command"=w357:enum16{"None", "Start Recal"}, "Data"=w359:u32)
        n124 = case shown="\"Start Recal\"" w357 {
          tunnel: w358 -> [w369 w373]
          tunnel: w365 -> [w370 w377]
          tunnel: [w370 w377] -> w364
          tunnel: [w369 w372] -> w363
          tunnel: w362 -> [_ _]
          tunnel: w361 -> [_ w374]
          tunnel: w359 -> [_ w371]
          tunnel: w358 -> [_ _]
          tunnel: ["Run" "Calibrate"] -> w356
          frame "None", Default {
          }
          frame "Start Recal" {
            n125 = Bundle By Name(cluster=w373, "ADIS16448DevRef.Calibration Time"=w371) -> (w372:T13)
            n126 = in-place {
              in-place-border: T15 {"Calibrated?"=FALSE, "IMU Detected?"=TRUE} ("element") -> [w378]
              n127 = in-place-dvr #6(w374) -> (w379:T21)  [unwired: 1 out]
              n128 = Bundle(cluster=w379, w378) -> (w380:T21)  [unwired: 4 in]
              n129 = in-place-dvr #6(w380) -> ()  [unwired: 2 out]
            }
          }
        }
      }
    }
  }
  n130 = Open VI Reference(vi path="Main Name") -> (vi reference=w9:refnum<vi>)  [unwired: 3 in, 3 out]
  n131 = while {
    tunnel: w9 -> [w382]
    tunnel: [w381] -> w3
    stop <- w381 stop-if-true
    n132 = property class="VI"(reference=w382) -> ("Exec.State"=w384:T26)  [unwired: 1 in, 2 out]
    n133 = Equal?(x=w384, y=T26."Idle" ("Execution:State")) -> (x = y?=w381:bool)
    n134 = Wait (ms)(milliseconds to wait=u32 250) -> ()  [unwired: 1 out]
  }
  n135 = flat-sequence {
    tunnel: w3 -> [_]
    frame #0 {
      n136 = call <vilib>:"WPI_DigitalOutputRefNum Registry Get.vi"("refnum name"="448 Status LED") -> ("error out"=w391:errorcluster, "DigitalOutputDevRef"=w390:T19)  [unwired: 9 in]
      n137 = call <vilib>:"WPI_DigitalOutputClose.vi"("error in (no error)"=w391, "DigitalOutputDevRef"=w390) -> ("error out"=w386:errorcluster)  [unwired: 9 in]
      n138 = call <vilib>:"WPI_SPIRefNum Registry Get.vi"("error in (no error)"=w386, "refnum name"="AutoSPI") -> ("error out"=w388:errorcluster, "SPIDevRef"=w387:T12)  [unwired: 8 in]
      n139 = call <vilib>:"WPI_SPIClose.vi"("error in (no error)"=w388, "SPIDevRef"=w387) -> ()  [unwired: 9 in, 1 out]
    }
    frame #1 {
      n140 = Stop() -> ()  [unwired: 1 in]
    }
  }
